vi "Execute Msg.vi"(7 "Actor in":refnum<class "Actor.lvclass">, 8 "Error in":errorcluster, 11 "TEMPLATE Msg in":refnum<class "TEMPLATE Msg.lvclass">) -> (0 "Error out":errorcluster, 2 "Msg Output":refnum<class "Msg Output.lvclass">, 5 "Actor out":refnum<class "Actor.lvclass">)   [LabVIEW 2025, in "_Template.lvlib" / "Templates.lvlib" / "TEMPLATE Msg.lvlib" / "TEMPLATE Msg.lvlib" / "TEMPLATE Msg.lvclass"]
uses:
  TEMPLATE Msg.lvclass
  TEMPLATE Msg.lvclass/TEMPLATE Msg.ctl
  TEMPLATE Msg Output/TEMPLATE Msg Output.lvlib
  TEMPLATE Msg Input/TEMPLATE Msg Input.lvlib
  TEMPLATE/TEMPLATE.lvclass
  jettl/jettl/Actor/Actor.lvclass
  jettl/jettl/Msg Output/Msg Output.lvclass
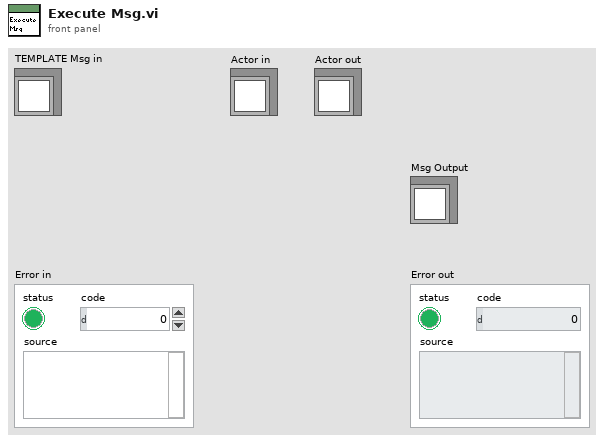
[diagram p1: front panel]
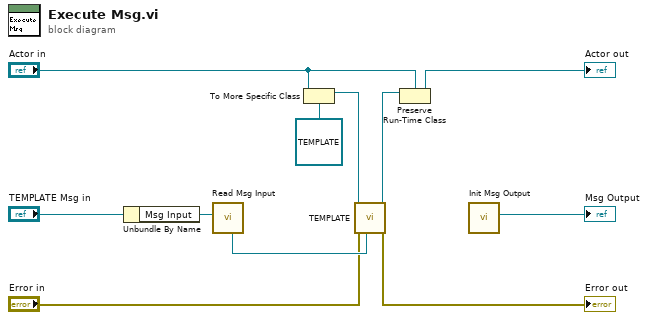
[diagram p0: block diagram]
diagram:
  n1 = Unbundle By Name("TEMPLATE Msg in") -> ("Msg Input"=w5:refnum<class "Msg Input.lvclass">)
  n2 = call "Read Msg Input.vi"("Msg Input"=w5) -> ("Teller"=w10:refnum<class "Teller.lvclass">)  [unwired: 9 in, 1 out]
  n3 = To More Specific Class(target class=refnum<class "TEMPLATE.lvclass"> refnum ("jettl Msg Template"), reference="Actor in") -> (specific class reference=w8:refnum<class "TEMPLATE.lvclass">)  [unwired: 1 in, 1 out]
  n4 = call-dynamic "TEMPLATE.vi"("Teller"=w10, "Error in"="Error in", "TEMPLATE in"=w8) -> ("Error out"=→"Error out":errorcluster, "TEMPLATE out"=w7:refnum<class "TEMPLATE.lvclass">)  [unwired: 7 in]
  n5 = Preserve Run-Time Class(object in=w7, 2:"Actor in") -> (object out=→"Actor out":refnum<class "Actor.lvclass">)  [unwired: 1 in, 1 out]
  n6 = call "Init Msg Output.vi"() -> ("Msg Output"=→"Msg Output":refnum<class "Msg Output.lvclass">)  [unwired: 11 in]
